vi "Bai1_3.vi"() -> ()   [LabVIEW 2018]
panel:
  out "RED":bool
  out "YELLOW":bool
  out "GREEN":bool
  out "RED 2":bool
  out "YELLOW  2":bool
  out "GREEN 2":bool
  out "RED 3":bool
  out "YELLOW  3":bool
  out "GREEN 3":bool
  out "RED 4":bool
  out "YELLOW  4":bool
  out "GREEN 4":bool
  out "Sogiay":i32
  in  "stop":bool
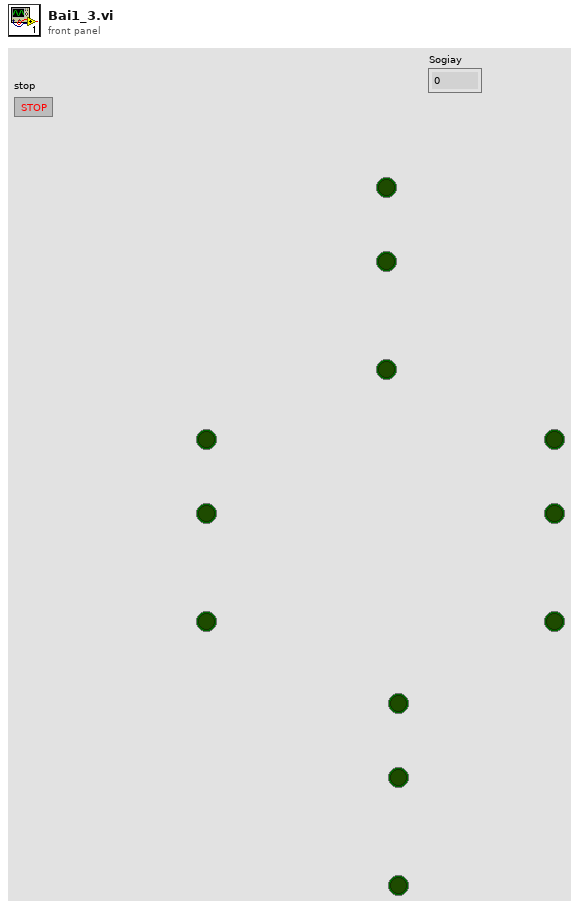
[diagram p1: front panel]
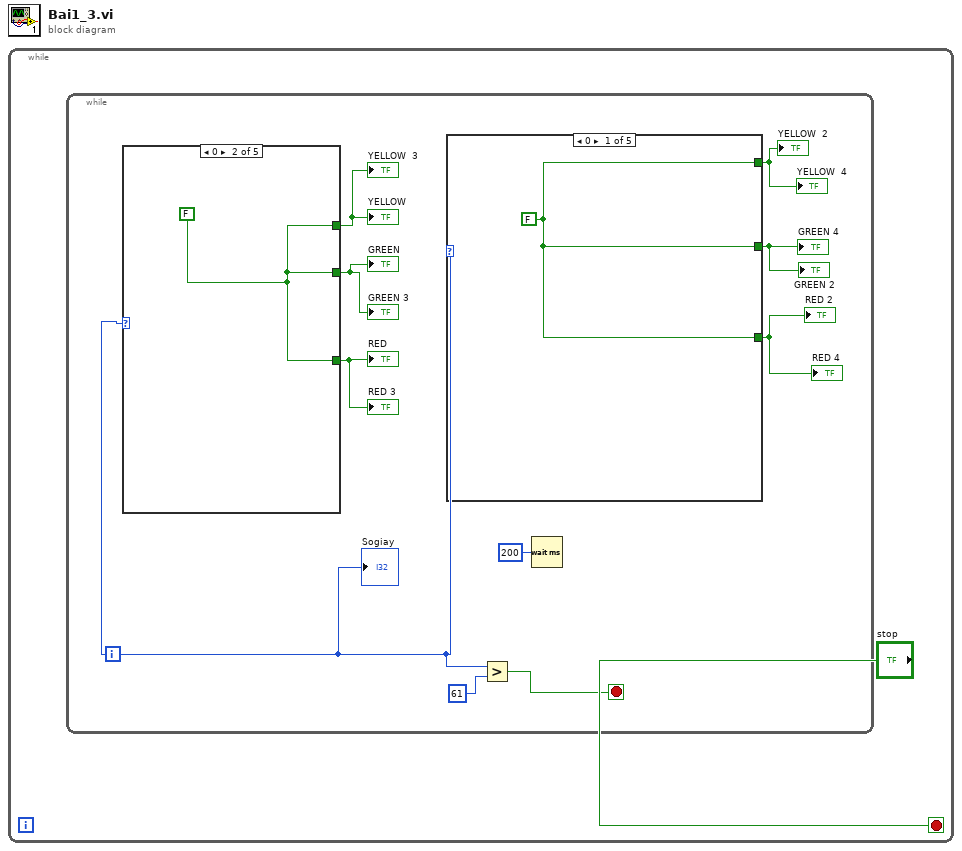
[diagram p0: block diagram]
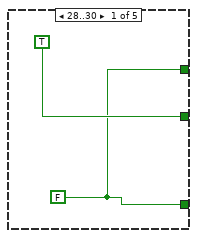
[diagram p2: hidden frame]
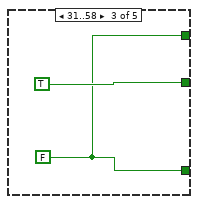
[diagram p3: hidden frame]
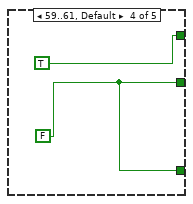
[diagram p4: hidden frame]
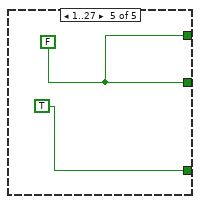
[diagram p5: hidden frame]
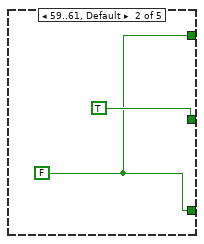
[diagram p6: hidden frame]
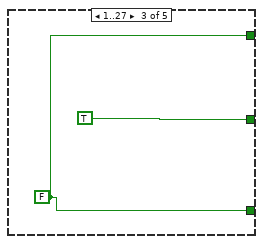
[diagram p7: hidden frame]
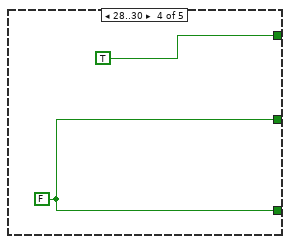
[diagram p8: hidden frame]
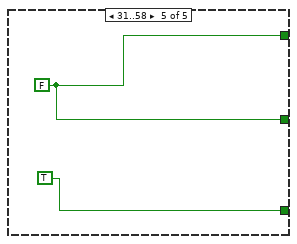
[diagram p9: hidden frame]
diagram:
  n1 = while {
    stop <- "stop" stop-if-true
    n2 = while {
      i -> [w2]
      stop <- w10 stop-if-true
      n3 = case shown="0" w2 {
        tunnel: [w12 w14 w15 TRUE ("YELLOW") w20] -> w5
        tunnel: [TRUE ("YELLOW  3") w14 TRUE ("YELLOW") w17 w20] -> w4
        tunnel: [w12 w14 w15 w17 TRUE ("YELLOW")] -> w3
        frame 28..30 {
          w12 = FALSE ("YELLOW")
        }
        frame 0 {
          w14 = FALSE ("YELLOW")
        }
        frame 31..58 {
          w15 = FALSE ("YELLOW")
        }
        frame 59..61, Default {
          w17 = FALSE ("YELLOW")
        }
        frame 1..27 {
          w20 = FALSE ("YELLOW")
        }
      }
      "RED" <- w3
      "YELLOW" <- w5
      "GREEN" <- w4
      "RED 3" <- w3
      "YELLOW  3" <- w5
      "GREEN 3" <- w4
      n4 = case shown="0" w2 {
        tunnel: [w21 TRUE ("YELLOW") TRUE w26 w28] -> w8
        tunnel: [w21 w22 w24 w26 TRUE] -> w6
        tunnel: [w21 w22 w24 TRUE w28] -> w7
        frame 0 {
          w21 = FALSE
        }
        frame 59..61, Default {
          w22 = FALSE ("YELLOW")
        }
        frame 1..27 {
          w24 = FALSE
        }
        frame 28..30 {
          w26 = FALSE
        }
        frame 31..58 {
          w28 = FALSE
        }
      }
      "RED 2" <- w6
      "YELLOW  2" <- w7
      "GREEN 2" <- w8
      "RED 4" <- w6
      "YELLOW  4" <- w7
      "GREEN 4" <- w8
      n5 = Greater?(x=w2, y=61) -> (0:w10:bool)
      n6 = Wait (ms)(milliseconds to wait=u32 200) -> ()  [unwired: 1 out]
      "Sogiay" <- w2
    }
  }
